vi "Read Error.vi"(8 "error in (no error)":errorcluster, 11 "Stability Data in":refnum<class "Stability Data.lvclass">) -> (0 "error out":errorcluster, 2 "Error":sgl, 3 "Stability Data out":refnum<class "Stability Data.lvclass">)   [LabVIEW 2015, in "Stability Data.lvclass"]
uses:
  Stability Data.lvclass
  Stability Data.lvclass/Stability Data.ctl
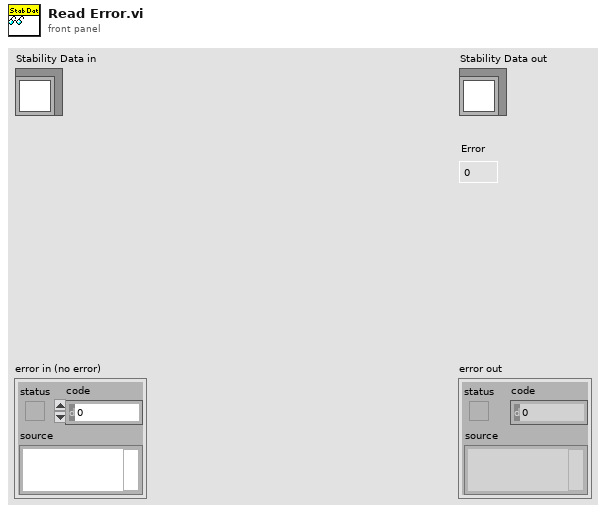
[diagram p1: front panel]
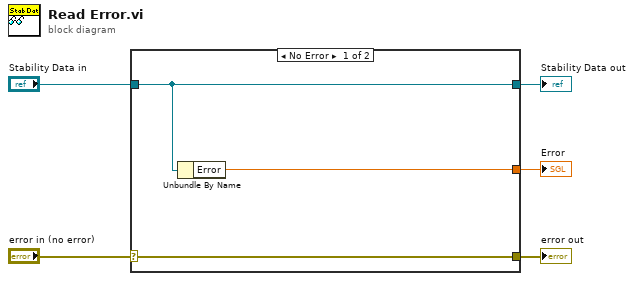
[diagram p0: block diagram]
diagram:
  n1 = case shown="No Error" "error in (no error)" {
    selector: "error in (no error)" -> [w8 w9]
    tunnel: [w8 w9] -> w4
    tunnel: [w7 w10] -> w2
    tunnel: "Stability Data in" -> [w7 w10]
    tunnel: [w6 _] -> w1
    frame No Error {
      n2 = Unbundle By Name(w7) -> ("Error"=w6:sgl)
    }
    frame Error {
    }
  }
  "error out" <- w4
  "Stability Data out" <- w2
  "Error" <- w1
